vi "Get Command Response.vi"(8 "error in (no error)":errorcluster, 10 "command":T4={"Command"=enum."Rx", "Parameters"={"arg1"=0, "arg2"=0}}, 11 "Dispatcher Interface in":refnum<class "Dispatcher Interface.lvclass">) -> (0 "error out":errorcluster, 1 "response expected?":bool, 2 "response":T1, 3 "Dispatcher Interface out":refnum<class "Dispatcher Interface.lvclass">)   [LabVIEW 2019, in "DSF Core.lvlib" / "Dispatcher Interface.lvclass"]
uses:
  Interface/Dispatcher/Dispatcher Interface.lvclass
  Interface/Dispatcher/Command Data.ctl
  Interface/Dispatcher/Command.ctl
  Interface/Dispatcher/Parameters.ctl
  Interface/Dispatcher/Response Data.ctl
  Interface/Dispatcher/Response.ctl
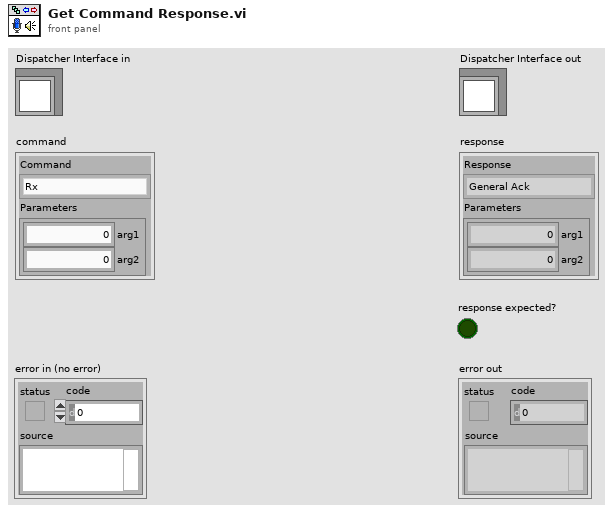
[diagram p1: front panel]
types:
  T1 = typedef "DSF Core.lvlib/Dispatcher Interface.lvclass/Response Data.ctl" = cluster{"Response":T2, "Parameters":T3}
  T2 = typedef "DSF Core.lvlib/Dispatcher Interface.lvclass/Response.ctl" = enum8{"General Ack", "Error", "Shutting Down"}
  T3 = typedef "DSF Core.lvlib/Dispatcher Interface.lvclass/Parameters.ctl" = cluster{"arg1":u64, "arg2":u64}
  T4 = typedef "DSF Core.lvlib/Dispatcher Interface.lvclass/Command Data.ctl" = cluster{"Command":T5, "Parameters":T3}
  T5 = typedef "DSF Core.lvlib/Dispatcher Interface.lvclass/Command.ctl" = enum8{"Idle", "Start", "Rx", "Tx", "Set Inline Buffer", "Shutdown", "Error"}
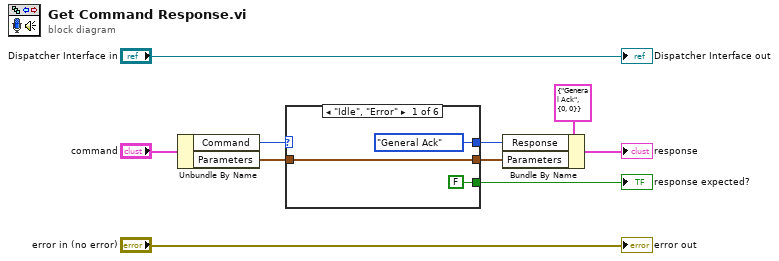
[diagram p0: block diagram]
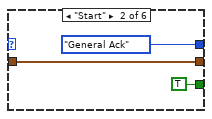
[diagram p2: hidden frame]
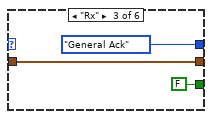
[diagram p3: hidden frame]
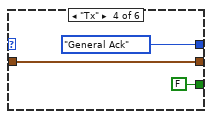
[diagram p4: hidden frame]
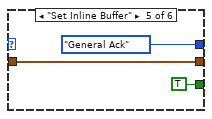
[diagram p5: hidden frame]
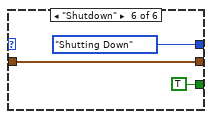
[diagram p6: hidden frame]
diagram:
  n1 = Unbundle By Name("command") -> ("Command"=w8:T5, "Parameters"=w7:T3)
  n2 = case shown="\"Idle\", \"Error\"" w8 {
    tunnel: w7 -> [w13 w15 w18 w22 w25 w28]
    tunnel: [Response."General Ack" ("Response") Response."General Ack" ("Response") Response."General Ack" ("Response") Response."General Ack" ("Response") Response."General Ack" ("Response") Response."Shutting Down" ("Response")] -> w5
    tunnel: [w13 w15 w18 w22 w25 w28] -> w4
    tunnel: [FALSE TRUE FALSE FALSE TRUE TRUE] -> w1
    frame "Idle", "Error" {
    }
    frame "Start" {
    }
    frame "Rx" {
    }
    frame "Tx" {
    }
    frame "Set Inline Buffer" {
    }
    frame "Shutdown" {
    }
  }
  "response expected?" <- w1
  n3 = Bundle By Name(cluster=T1 {"Response"=enum."General Ack", "Parameters"={"arg1"=0, "arg2"=0}} ("Dispatcher Response"), "Response"=w5, "Parameters"=w4) -> (→"response":T1)
  "error out" <- "error in (no error)"
  "Dispatcher Interface out" <- "Dispatcher Interface in"
